vi "GetNextProcessModule.vi"   [LabVIEW 2017, in "FileFlow.lvlib"]
doc: "Transfers an in-memory TDMS file to the message queue for the next process in the Fileflow Script. This VI looks up which process is next in order based on the value of the <B>source</B> input. If the <B>source</B> is the final process in the Fileflow Script, this VI sends a SendTDMSFileinMemory message to the File Manager process. File Manager manages complete files until they are transferred to the server."
uses:
  <vilib>/addons/InsightCM/Devices/Shared/Common/FileFlow/FileFlow.lvlib
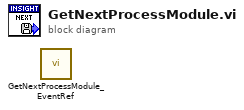
[diagram p0: block diagram]
diagram:
  n1 = call <vilib>:"GetNextProcessModule_EventRef.vi"() -> ()  [unwired: 10 in, 2 out]
